vi "csmdoc-Populate Single Example Description.vi"(6 "Show FP":bool, 8 "error in (no error)":errorcluster, 10 "VI Description":string, 11 "Path":path) -> (0 "error out":errorcluster)   [LabVIEW 2017, in "csmdoc.lvlib"]
uses:
  csmdoc.lvlib
  _Shared/CSM Shared.lvlib
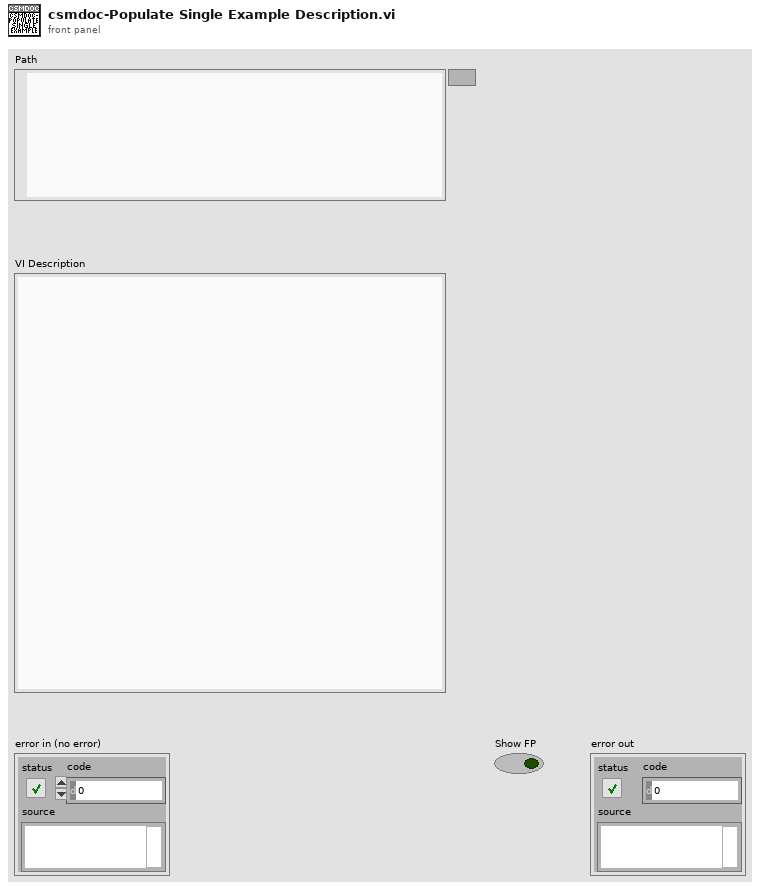
[diagram p1: front panel]
types:
  T1 = typedef "csmdoc.lvlib/DocElement.ctl" = cluster{"ID":string, "Content":string[], "SubIDs":string[], "Path":string[]}
  T2 = typedef "csmdoc.lvlib/DocNote.ctl" = cluster{"ID":string, "Content":string, "Type":string}
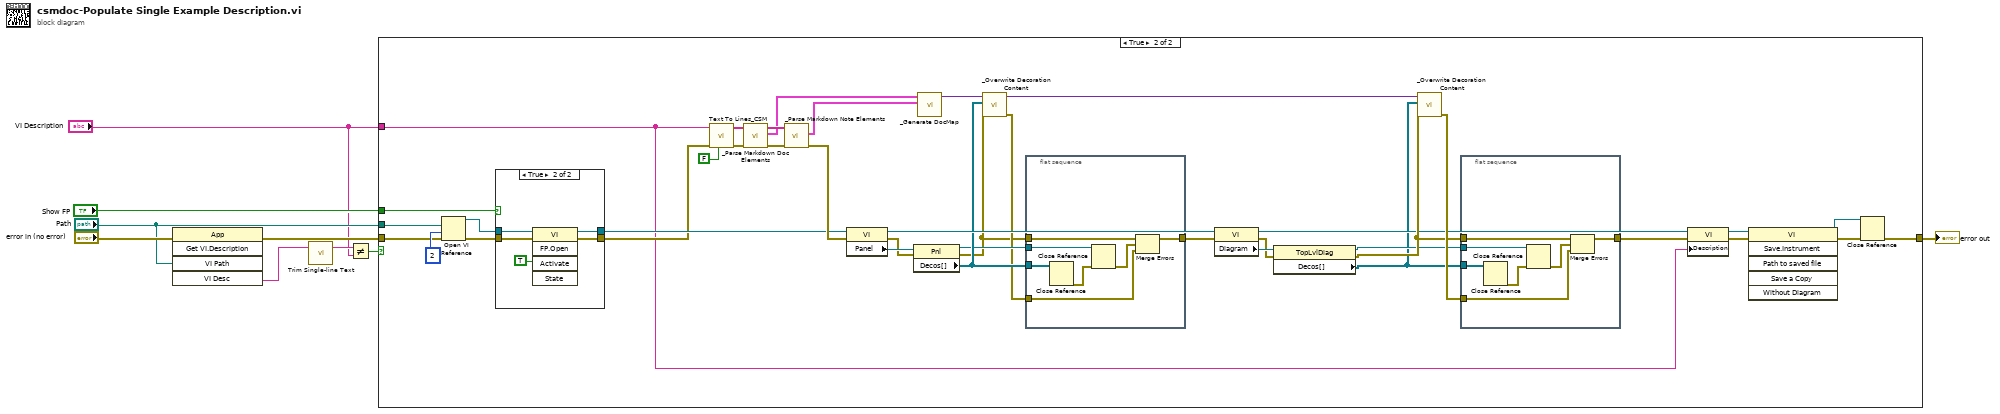
[diagram p0: block diagram]
diagram:
  n1 = invoke class="App" method="Get VI.Description"(error in="error in (no error)", "VI Path"="Path") -> (error out=w9:errorcluster, "VI Desc"=w3:string)  [unwired: 3 in, 3 out]
  n2 = call "Trim Single-line Text.vi"("single-line text"=w3) -> ("trimed text"=w7:string)  [unwired: 2 in]
  n3 = Not Equal?(x=w7, y="VI Description") -> (x != y?=w8:bool)
  n4 = case shown="True" w8 {
    tunnel: w9 -> [w10 w46]
    tunnel: "VI Description" -> [_ w24]
    tunnel: [w10 w43] -> w5
    tunnel: "Show FP" -> [_ w50]
    tunnel: "Path" -> [_ w42]
    frame False {
    }
    frame True {
      n5 = Open VI Reference(vi path=w42, options=2, error in (no error)=w46) -> (vi reference=w47:refnum<vi>, error out=w48:errorcluster)  [unwired: 3 in]
      n6 = case shown="True" w50 {
        tunnel: w48 -> [w65 w70]
        tunnel: w47 -> [w66 w69]
        tunnel: [w65 w68] -> w25
        tunnel: [w66 w67] -> w26
        frame False {
        }
        frame True {
          n7 = invoke class="VI" method="FP.Open"(reference=w69, error in=w70, "Activate"=TRUE ("Activate?")) -> (reference out=w67:refnum<vi>, error out=w68:errorcluster)  [unwired: 2 in, 3 out]
        }
      }
      n8 = call "Text To Lines_CSM.vi"("Remove Empty Lines? (T)"=FALSE ("Remove Empty Lines?(T)"), "error in (no error)"=w25, "String"=w24) -> ("error out"=w39:errorcluster, "Lines"=w40:string[])  [unwired: 7 in]
      n9 = call "_Parse Markdown Doc Elements.vi"("Error in"=w39, "Lines"=w40) -> ("Error out"=w35:errorcluster, "Array"=w33:T1[], "Lines (dup)"=w36:string[])  [unwired: 7 in]
      n10 = call "_Parse Markdown Note Elements.vi"("Error in"=w35, "Lines"=w36) -> ("Error out"=w34:errorcluster, "Array"=w32:T2[])  [unwired: 7 in, 1 out]
      n11 = property class="VI"(reference=w26, error in=w34) -> (reference out=w37:refnum<vi>, error out=w28:errorcluster, "Panel"=w38:refnum<vi>)
      n12 = property class="Pnl"(reference=w38, error in=w28) -> (reference out=w30:refnum<vi>, error out=w22:errorcluster, "Decos[]"=w31:refnum<vi>[])
      n13 = call "_Generate DocMap.vi"("Array 2"=w32, "Array"=w33) -> ("Variant"=w27:variant)  [unwired: 9 in]
      n14 = call "_Overwrite Decoration Content.vi"("error in (no error)"=w22, "Decos[]"=w31, "Variant in"=w27) -> ("error out"=w23:errorcluster, "Variant out"=w16:variant)  [unwired: 7 in]
      n15 = flat-sequence {
        tunnel: w31 -> [w64]
        tunnel: w30 -> [w63]
        tunnel: [w61] -> w29
        tunnel: w22 -> [w59]
        tunnel: w23 -> [w58]
        frame #0 {
          n16 = Close Reference(reference=w64) -> (error out=w62:errorcluster)  [unwired: 1 in]
          n17 = Close Reference(reference=w63, error in (no error)=w62) -> (error out=w60:errorcluster)
          n18 = Merge Errors(w59, w60, w58) -> (w61:errorcluster)
        }
      }
      n19 = property class="VI"(reference=w37, error in=w29) -> (reference out=w15:refnum<vi>, error out=w20:errorcluster, "Diagram"=w21:refnum<vi>)
      n20 = property class="TopLvlDiag"(reference=w21, error in=w20) -> (reference out=w17:refnum<vi>, error out=w18:errorcluster, "Decos[]"=w13:refnum<vi>[])
      n21 = call "_Overwrite Decoration Content.vi"("error in (no error)"=w18, "Decos[]"=w13, "Variant in"=w16) -> ("error out"=w19:errorcluster)  [unwired: 7 in, 1 out]
      n22 = flat-sequence {
        tunnel: w13 -> [w57]
        tunnel: w17 -> [w56]
        tunnel: [w54] -> w14
        tunnel: w18 -> [w52]
        tunnel: w19 -> [w51]
        frame #0 {
          n23 = Close Reference(reference=w57) -> (error out=w55:errorcluster)  [unwired: 1 in]
          n24 = Close Reference(reference=w56, error in (no error)=w55) -> (error out=w53:errorcluster)
          n25 = Merge Errors(w52, w53, w51) -> (w54:errorcluster)
        }
      }
      n26 = property class="VI"(reference=w15, error in=w14, "Description"=w24) -> (reference out=w11:refnum<vi>, error out=w12:errorcluster)
      n27 = invoke class="VI" method="Save.Instrument"(reference=w11, error in=w12) -> (reference out=w44:refnum<vi>, error out=w45:errorcluster)  [unwired: 4 in, 4 out]
      n28 = Close Reference(reference=w44, error in (no error)=w45) -> (error out=w43:errorcluster)
    }
  }
  "error out" <- w5
